vi "Generate Simulated Data.vi"(8 "error in (no error)":errorcluster, 11 "Channel Settings":T1[](array[typedef])) -> (0 "error out":errorcluster, 2 "Graph Data":T3)   [LabVIEW 2021, in "Acquisition.lvlib"]
doc: "Generate a separate waveform for each channel in 'Channel Settings'."
uses:
  Acquisition.lvlib
  controls/Acquired Data.ctl
  Channel Settings.ctl
  IO Device.ctl
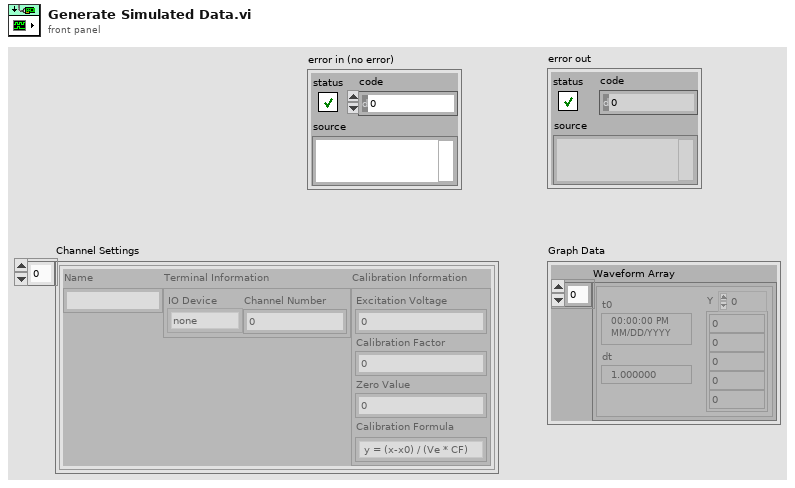
[diagram p1: front panel]
types:
  T1 = typedef "Acquisition.lvlib/Channel Settings.ctl" = cluster{"Name":string, "Terminal Information":cluster{"IO Device":T2, "Channel Number":i32}, "Calibration Information":cluster{"Excitation Voltage":dbl, "Calibration Factor":dbl, "Zero Value":dbl, "Calibration Formula":string}}
  T2 = typedef "Acquisition.lvlib/IO Device.ctl" = enum16{"none", "9219", "9401"}
  T3 = typedef "Acquired Data.ctl" = cluster{"Waveform Array":waveform(dbl)[]}
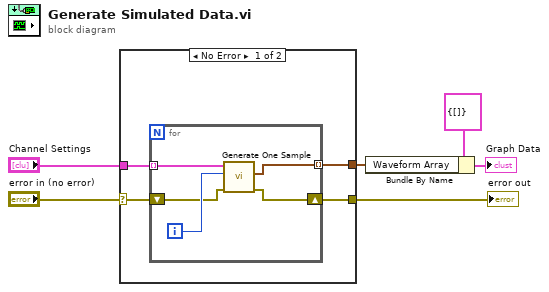
[diagram p0: block diagram]
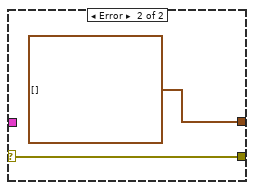
[diagram p2: hidden frame]
diagram:
  n1 = case shown="No Error" "error in (no error)" {
    selector: "error in (no error)" -> [w9 w17]
    tunnel: [w10 w17] -> w5
    tunnel: "Channel Settings" -> [w8 _]
    tunnel: [w7 waveform(dbl)[] []] -> w1
    frame No Error {
      n2 = for {
        shift-right: [w15] -> w10
        shift-left: w9 -> [w12]
        tunnel: w8 -> [w14] mode=indexing
        tunnel: [w11] -> w7 mode=indexing
        i -> [w13]
        n3 = call "Generate One Sample.vi"("error in (no error)"=w12, "Active channel index"=w13, "Channel Settings"=w14) -> ("error out"=w15:errorcluster, "Waveform"=w11:waveform(dbl))  [unwired: 7 in]
      }
    }
    frame Error {
    }
  }
  "error out" <- w5
  n4 = Bundle By Name(cluster=T3 {"Waveform Array"=[]} ("Acquired Data"), "Waveform Array"=w1) -> (→"Graph Data":T3)
